vi "CfgManager Test Launcher.vi"() -> ()   [LabVIEW 2013]
uses:
  Cache/ConfigManager.Cache.lvclass
  Manager/ConfigManager.lvclass
panel:
  out "keys listed":string[](array[string])
  out "keys written":string[](array[string])
  out "Values":variant[](array[variant])
  out "keys read":string[](array[string])
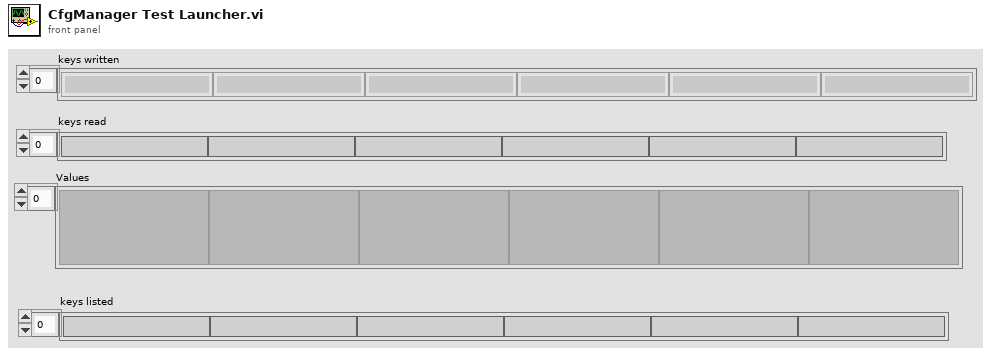
[diagram p1: front panel]
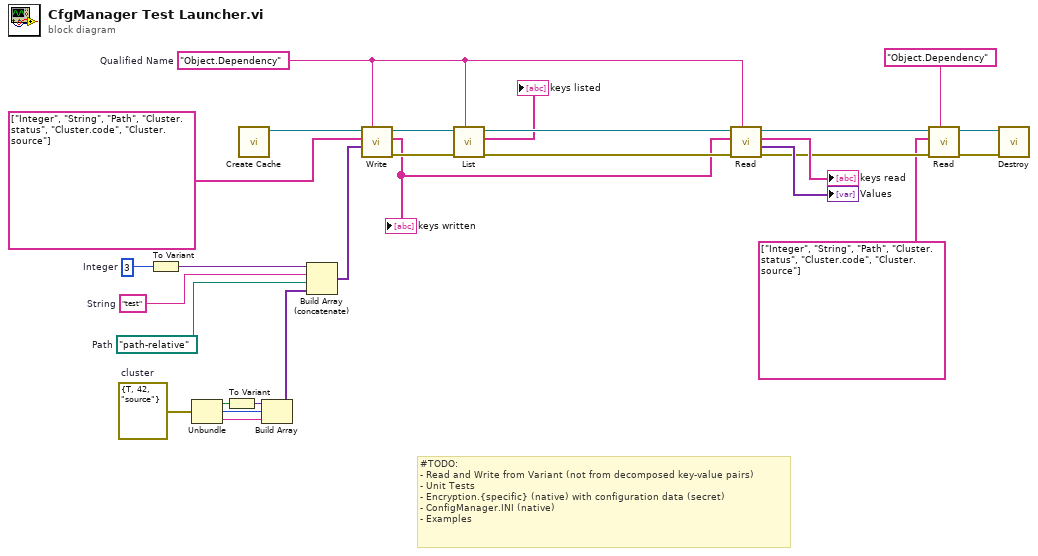
[diagram p0: block diagram]
diagram:
  w16 = "Object.Dependency"  # Qualified Name
  w6 = errorcluster {"status"=TRUE, "code"=42, "source"="source"}  # cluster
  w22 = path "path-relative"  # Path
  w23 = "test"  # String
  w25 = 3  # Integer
  # "#TODO: \n- Read and Write from Variant (not from decomposed key-value pairs)\n- Unit Tests\n- Encryption.{specific} (native) with configuration data (secret)\n- ConfigManager.INI (native)\n- Examples"
  n1 = To Variant(anything=w25) -> (Variant=w24:variant)
  n2 = Unbundle(w6) -> ("status"=w5:bool, "code"=w4:i32, "source"=w3:string)
  n3 = To Variant(anything=w5) -> (Variant=w2:variant)
  n4 = call "Create Cache.vi"() -> ("ConfigManager.Cache"=w26:refnum<class "ConfigManager.Cache.lvclass">)  [unwired: 11 in]
  n5 = Build Array(w2, w4, w3) -> (w1:variant[])
  n6 = Build Array (concatenate)(w24, w23, w22, w1) -> (w21:variant[])
  n7 = call "Write.vi"("Qualified Name"=w16, "Values"=w21, "keys"=string[] ["Integer", "String", "Path", "Cluster.status", "Cluster.code", "Cluster.source"] ("keys written"), "ConfigManager in"=w26) -> ("error out"=w18:errorcluster, "keys dup"=w13:string[], "ConfigManager out"=w20:refnum<class "ConfigManager.Cache.lvclass">)  [unwired: 5 in]
  "keys written" <- w13
  n8 = call "List.vi"("Qualified Name"=w16, "error in (no error)"=w18, "ConfigManager in"=w20) -> ("error out"=w17:errorcluster, "Keys"=→"keys listed":string[], "ConfigManager out"=w19:refnum<class "ConfigManager.Cache.lvclass">)  [unwired: 6 in]
  n9 = call "Read.vi"("Qualified Name"=w16, "error in (no error)"=w17, "keys in"=w13, "ConfigManager in"=w19) -> ("error out"=w10:errorcluster, "Values"=→"Values":variant[], "keys"=→"keys read":string[], "ConfigManager out"=w12:refnum<class "ConfigManager.Cache.lvclass">)  [unwired: 4 in]
  n10 = call "Read.vi"("Qualified Name"="Object.Dependency" ("Name"), "error in (no error)"=w10, "keys in"=string[] ["Integer", "String", "Path", "Cluster.status", "Cluster.code", "Cluster.source"] ("keys written"), "ConfigManager in"=w12) -> ("error out"=w9:errorcluster, "ConfigManager out"=w11:refnum<class "ConfigManager.Cache.lvclass">)  [unwired: 4 in, 2 out]
  n11 = call-dynamic "Destroy.vi"("error in (no error)"=w9, "ConfigManager.Cache in"=w11) -> ()  [unwired: 8 in, 2 out]
